vi "Write port.vi"(8 "error in (no error)":errorcluster, 10 "port":i32, 11 "MelsecTCP in":refnum<class "InovanceTCP.lvclass">) -> (0 "error out":errorcluster, 3 "MelsecTCP out":refnum<class "InovanceTCP.lvclass">)   [LabVIEW 2020, in "HslCommunication.lvlib" / "InovanceTCP.lvclass"]
uses:
  InovanceTCP.lvclass
  InovanceTCP.lvclass/InovanceTCP.ctl
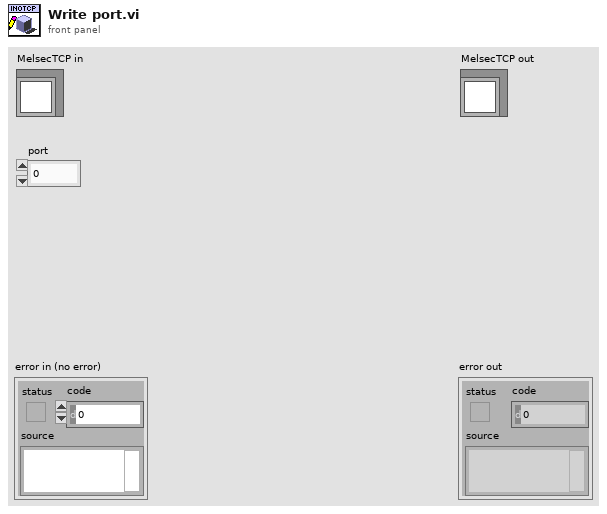
[diagram p1: front panel]
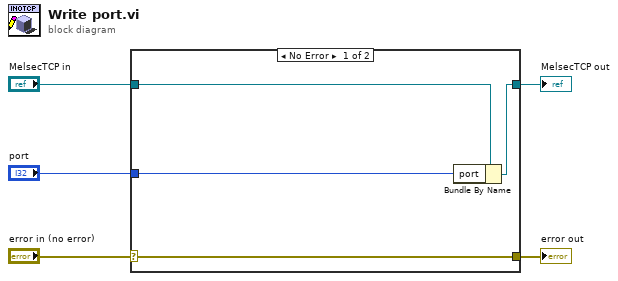
[diagram p0: block diagram]
diagram:
  n1 = case shown="No Error" "error in (no error)" {
    selector: "error in (no error)" -> [w9 w10]
    tunnel: [w9 w10] -> w4
    tunnel: [w7 w11] -> w2
    tunnel: "MelsecTCP in" -> [w8 w11]
    tunnel: "port" -> [w6 _]
    frame No Error {
      n2 = Bundle By Name(cluster=w8, "port"=w6) -> (w7:refnum<class "InovanceTCP.lvclass">)
    }
    frame Error {
    }
  }
  "error out" <- w4
  "MelsecTCP out" <- w2
